vi "Database-SQLiteGetActiveConn.vi"(7 "PageID":string, 8 "error in (no error)":errorcluster, 11 "Database-Actor in":refnum<class "Database-Actor.lvclass">) -> (0 "error out":errorcluster, 2 "Active Plugin Caller":refnum<class "FTW-ActorConnector.lvclass">, 3 "Database-Actor out":refnum<class "Database-Actor.lvclass">)   [LabVIEW 2013]
uses:
  ftw-dataflow/Core/utils/CodeGen/SQLite-Fetch/FTW-SQLite-Fetch.xnode
  ftw-dataflow/Actor/src/Connector/FTW-ActorConnector.lvclass
  ftw-dataflow/Core/src/Database/FTW-SQLite-PrepareStatement.vi
  ftw-dataflow/Core/src/Database/FTW-SQLite-Connector.lvclass
  ftw-dataflow/Core/src/Database/FTW-SQLite-LibraryReturnValue.vi
  ftw-dataflow/Core/src/Error/FTW-ERR-StatusOK.vi
  ftw-dataflow/Core/src/Error/FTW-ERR-ThrowImpossibleError.vi
  ftw-dataflow/Core/src/Database/FTW-SQLite-LibraryFilepath.vi
  ftw-dataflow/Core/src/Time/FTW-Time-Uptime.vi
  Database-Actor.lvclass
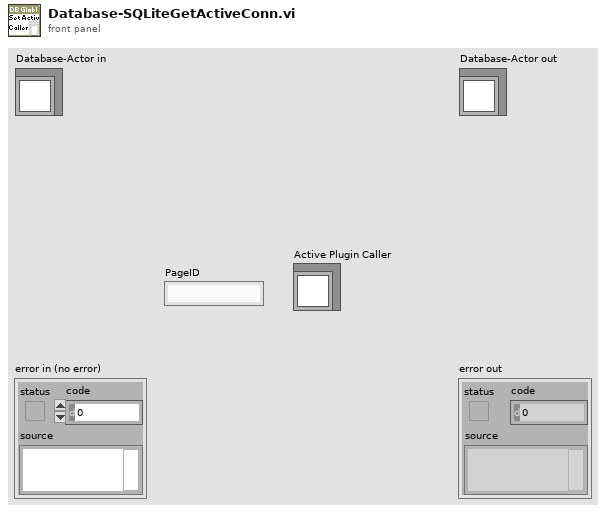
[diagram p1: front panel]
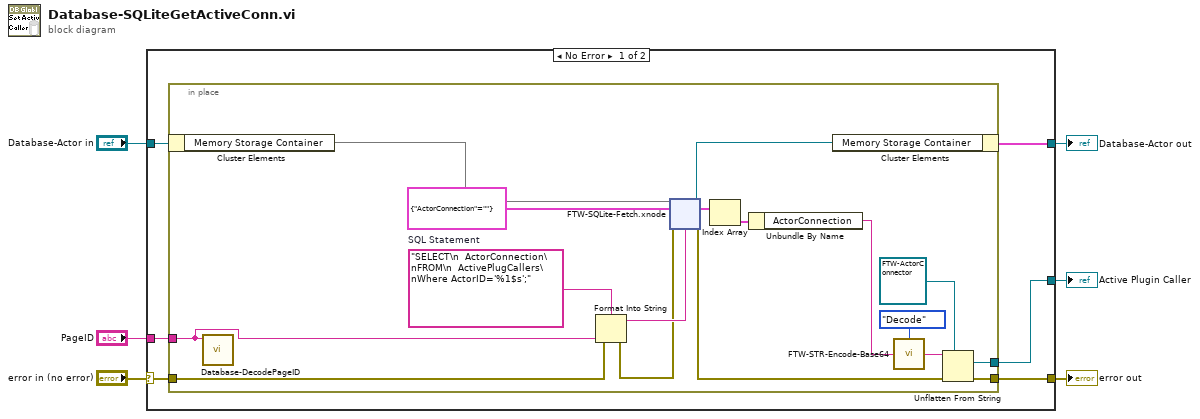
[diagram p0: block diagram]
diagram:
  n1 = case shown="No Error" "error in (no error)" {
    selector: "error in (no error)" -> [w8 w143]
    tunnel: [w7 w143] -> w5
    tunnel: [w10 w142] -> w3
    tunnel: "Database-Actor in" -> [w11 w142]
    tunnel: [w12 _] -> w2
    tunnel: "PageID" -> [w9 _]
    frame No Error {
      n2 = in-place {
        in-place-border: w8 -> [w19]
        in-place-border: [w18] -> w7
        in-place-border: w9 -> [w13]
        in-place-border: [w14] -> w12
        w28 = "SELECT\n  ActorConnection\nFROM\n  ActivePlugCallers\nWhere ActorID='%1$s';"  # SQL Statement
        n3 = in-place-cluster #1(w11) -> ("Memory Storage Container"=w29)
        n4 = call "Database-DecodePageID.vi"("PageID"=w13) -> ()  [unwired: 10 in, 1 out]
        n5 = Format Into String(format string=w28, error in=w19, w13) -> (resulting string=w27:string, error out=w17:errorcluster)  [unwired: 1 in]
        n6 = xnode "FTW-SQLite-Fetch.xnode"("SQLite Connector"=w29, "SQL Script"=w27, "Row Datatype"=cluster{"ActorConnection":string} {"ActorConnection"=""}, "error in"=w17) -> ("SQLite Connector out"=w26:refnum<class "FTW-SQLite-Connector.lvclass">, "Result Set"=w23:cluster{"ActorConnection":string}[], "error out"=w16:errorcluster)  [unwired: 2 out]
        n7 = Index Array(array=w23) -> (element=w22:cluster{"ActorConnection":string})  [unwired: 1 in]
        n8 = Unbundle By Name(w22) -> ("ActorConnection"=w21:string)
        n9 = in-place-cluster #1("Memory Storage Container"=w26) -> (w10:cluster{})
        n10 = call "FTW-STR-Encode-Base64.vi"("Input"=w21, "Direction"=enum16{"Encode", "Decode"}."Decode") -> ("Output"=w20:string)
        n11 = Unflatten From String(type=refnum<class "FTW-ActorConnector.lvclass"> refnum ("Plugin Caller"), binary string=w20, error in (no error)=w16) -> (value=w14:refnum<class "FTW-ActorConnector.lvclass">, error out=w18:errorcluster)  [unwired: 2 in, 1 out]
      }
    }
    frame Error {
    }
  }
  "error out" <- w5
  "Database-Actor out" <- w3
  "Active Plugin Caller" <- w2
